vi "Parse Elements Treewise.vi"(6 "VI Refs":refnum<vi>[](array[refnum]), 7 "VI Data in":T3[](array[typedef]), 8 "error in":errorcluster, 9 "Parents":string[](array[string]), 10 "XML Info":T2, 11 "Node in":refnum<k20>) -> (0 "error out":errorcluster, 3 "Node out":refnum<k20>, 4 "VI Refs out":refnum<vi>[](array[refnum]), 5 "VI Data out":T3[](array[typedef]))   [LabVIEW 2020, in "VI Properties Editor.lvlib"]
uses:
  VI Properties Editor.lvlib
  <vilib>/xml/NI_XML.lvlib
  <vilib>/xml/Close Reference(Node).vi
  CTLs/XPath Get Attribute.ctl
  <vilib>/picture/picture.llb/imagedata.ctl
  CTLs/VI Properties.ctl
  CTLs/Control Properties.ctl
  CTLs/VI Data.ctl
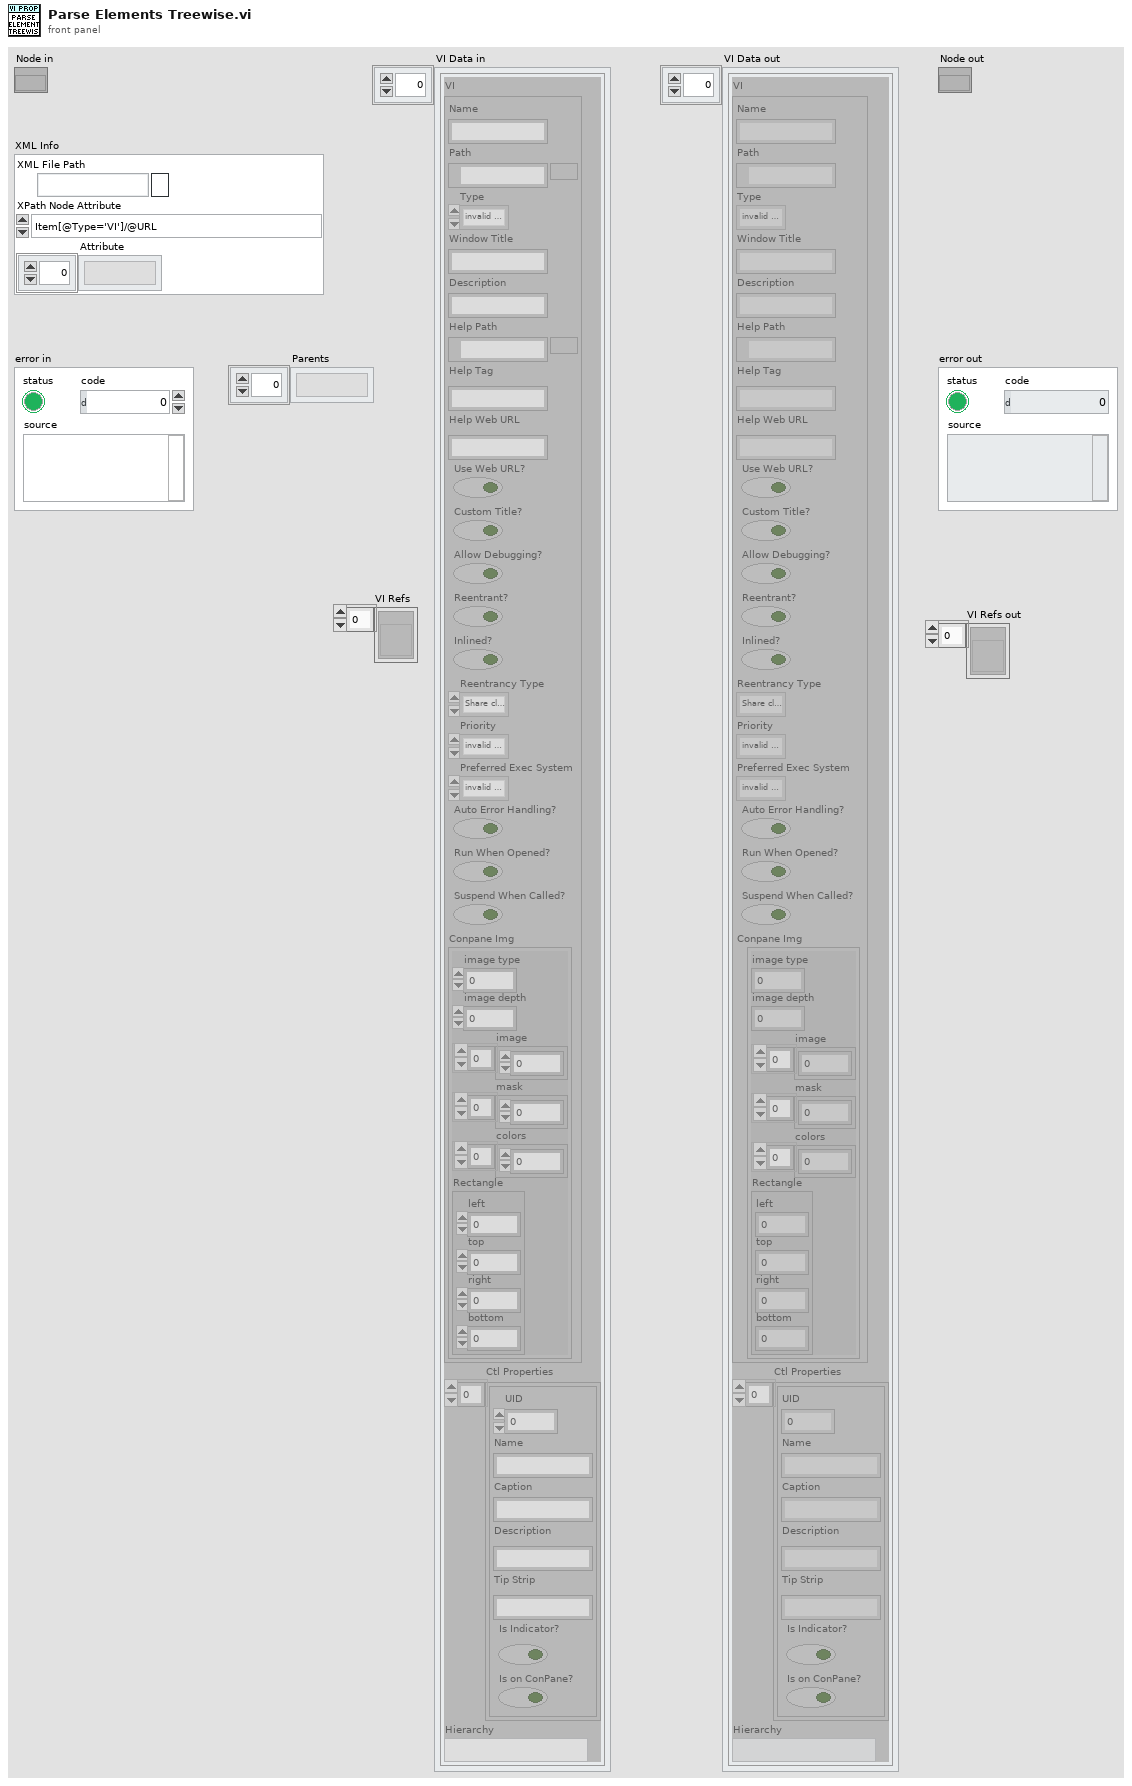
[diagram p1: front panel]
types:
  T1 = typedef "VI Properties Editor.lvlib/XPath Get Attribute.ctl" = enum16{"Item[@Type='VI']/@URL", "Item[@Type='LVClass']/@URL", "Item[@Type='Library']/@URL", "Item[@Type='Folder' and not (@URL)]/@Name", "@Name"}
  T2 = cluster{"XML File Path":path, "XPath Node Attribute":T1, "Attribute":string[]}
  T3 = typedef "VI Properties Editor.lvlib/VI Data.ctl" = cluster{"VI":T4, "Ctl Properties":T6[], "Hierarchy":string}
  T4 = typedef "VI Properties Editor.lvlib/VI Properties.ctl" = cluster{"Name":string, "Path":path, "Type":enum32{"invalid VI type", "Standard VI", "Control VI", "Global VI", "Polymorphic VI", "Configuration VI", "SubSystem", "Facade VI", "Method VI", "Statechart Diagram VI"}, "Window Title":string, "Description":string, "Help Path":path, "Help Tag":string, "Help Web URL":string, "Use Web URL?":bool, "Custom Title?":bool, "Allow Debugging?":bool, "Reentrant?":bool, "Inlined?":bool, "Reentrancy Type":enum16{"Share clones between instances", "Preallocate clone for each instance"}, "Priority":enum32{"invalid priority", "background priority", "normal priority", "above normal priority", "high priority", "time critical priority", "subroutine"}, "Preferred Exec System":enum32{"invalid execution system", "user interface", "standard", "instrument i/o", "data acquisition", "other 1", "other 2", "same as caller"}, "Auto Error Handling?":bool, "Run When Opened?":bool, "Suspend When Called?":bool, "Conpane Img":T5}
  T5 = typedef "imagedata.ctl" = cluster{"image type":i32, "image depth":i32, "image":u8[], "mask":u8[], "colors":u32[], "Rectangle":cluster{"left":i16, "top":i16, "right":i16, "bottom":i16}}
  T6 = typedef "VI Properties Editor.lvlib/Control Properties.ctl" = cluster{"UID":i32, "Name":string, "Caption":string, "Description":string, "Tip Strip":string, "Is Indicator?":bool, "Is on ConPane?":bool}
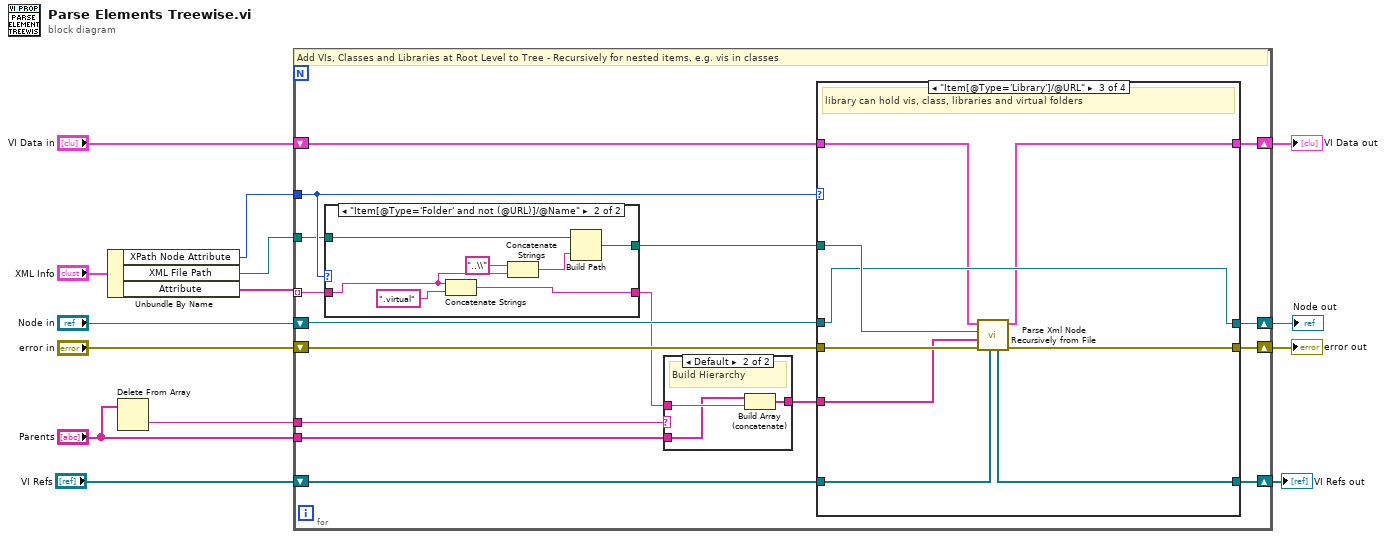
[diagram p0: block diagram]
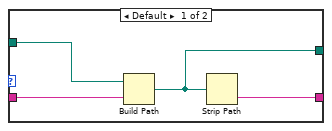
[diagram p2: hidden frame]
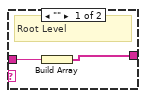
[diagram p3: hidden frame]
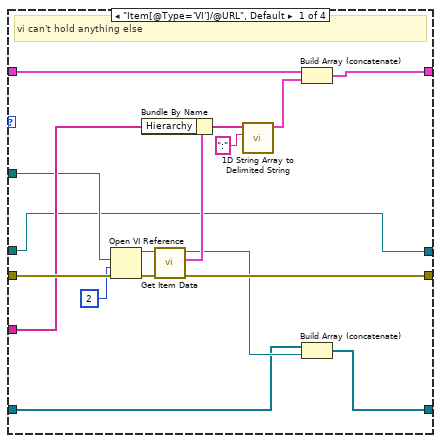
[diagram p4: hidden frame]
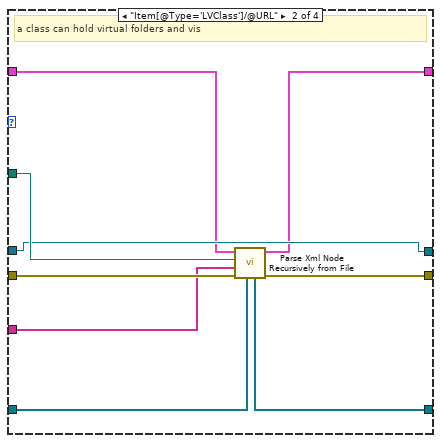
[diagram p5: hidden frame]
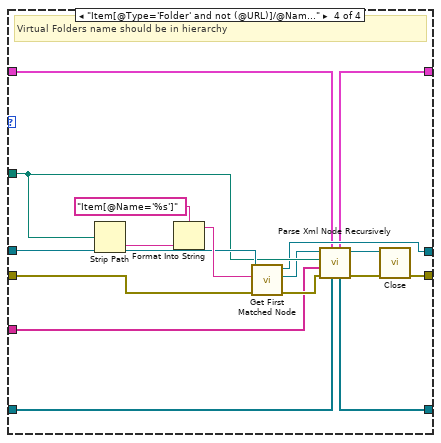
[diagram p6: hidden frame]
diagram:
  n1 = Unbundle By Name("XML Info") -> ("XPath Node Attribute"=w4:T1, "XML File Path"=w5:path, "Attribute"=w3:string[])
  n2 = Delete From Array(array="Parents") -> (deleted portion=w8:string)  [unwired: 2 in, 1 out]
  n3 = for {
    shift-right: [w30] -> w10
    shift-left: "error in" -> [w24]
    tunnel: w4 -> [w22]
    tunnel: w5 -> [w19]
    tunnel: w3 -> [w20] mode=indexing
    tunnel: "Parents" -> [w25]
    shift-right: [w28] -> w13
    shift-left: "VI Data in" -> [w27]
    tunnel: w8 -> [w26]
    shift-right: [w17] -> w7
    shift-left: "Node in" -> [w23]
    shift-right: [w15] -> w1
    shift-left: "VI Refs" -> [w16]
    # "Add VIs, Classes and Libraries at Root Level to Tree - Recursively for nested items, e.g. vis in classes"
    n4 = case shown="\"Item[@Type='Folder' and not (@URL)]/@Name\"" w22 {
      tunnel: w20 -> [w33 w39]
      tunnel: [w32 w40] -> w21
      tunnel: w19 -> [w34 w37]
      tunnel: [w31 w35] -> w18
      frame Default {
        n5 = Build Path(base path=w34, name or relative path=w33) -> (appended path=w31:path)
        n6 = Strip Path(path=w31) -> (name=w32:string)  [unwired: 1 out]
      }
      frame "Item[@Type='Folder' and not (@URL)]/@Name" {
        # "Virtual F."
        n7 = Concatenate Strings(w39, ".virtual" ("string")) -> (w40:string)
        n8 = Concatenate Strings("..\\" ("string"), w39) -> (w36:string)
        n9 = Build Path(base path=w37, name or relative path=w36) -> (appended path=w35:path)
      }
    }
    n10 = case shown="Default" w26 {
      tunnel: w21 -> [w43 w46]
      tunnel: [w42 w45] -> w29
      tunnel: w25 -> [_ w44]
      frame "" {
        # "Root Level"
        n11 = Build Array(w43) -> (w42:string[])
      }
      frame Default {
        # "Build Hierarchy"
        n12 = Build Array (concatenate)(w44, w46) -> (w45:string[])
      }
    }
    n13 = case shown="\"Item[@Type='Library']/@URL\"" w22 {
      tunnel: [w63 w72 w80 w97] -> w30
      tunnel: w24 -> [w62 w71 w81 w93]
      tunnel: w18 -> [w51 w70 w79 w91]
      tunnel: w29 -> [w57 w69 w78 w86]
      tunnel: [w52 w66 w75 w84] -> w28
      tunnel: w27 -> [w56 w67 w76 w85]
      tunnel: w23 -> [w50 w68 w77 w94]
      tunnel: [w50 w68 w77 w87] -> w17
      tunnel: w16 -> [w48 w65 w74 w83]
      tunnel: [w47 w64 w73 w82] -> w15
      frame "Item[@Type='VI']/@URL", Default {
        # "vi can't hold anything else"
        n14 = Open VI Reference(vi path=w51, options=2, error in (no error)=w62) -> (vi reference=w60:refnum<vi>, error out=w61:errorcluster)  [unwired: 3 in]
        n15 = call "Get Item Data.vi"("error in (no error)"=w61, "VI Ref"=w60) -> ("error out"=w63:errorcluster, "VI Data"=w55:T3, "VI Ref out"=w49:refnum<vi>)  [unwired: 7 in]
        n16 = call <vilib>:"1D String Array to Delimited String.vi"("delimiter"=":", "string array"=w57) -> ("delimited string"=w53:string)  [unwired: 9 in]
        n17 = Bundle By Name(cluster=w55, "Hierarchy"=w53) -> (w54:T3)
        n18 = Build Array (concatenate)(w56, w54) -> (w52:T3[])
        n19 = Build Array (concatenate)(w48, w49) -> (w47:refnum<vi>[])
      }
      frame "Item[@Type='LVClass']/@URL" {
        # "a class can hold virtual folders and vis"
        n20 = call "Parse Xml Node Recursively from File.vi"("VI Refs"=w65, "error in"=w71, "Parents"=w69, "Path to XML document"=w70, "VI Data"=w67) -> ("error out"=w72:errorcluster, "VI Data out"=w66:T3[], "VI Refs out"=w64:refnum<vi>[])  [unwired: 4 in]
      }
      frame "Item[@Type='Library']/@URL" {
        # "library can hold vis, class, libraries and virtual folders"
        n21 = call "Parse Xml Node Recursively from File.vi"("VI Refs"=w74, "error in"=w81, "Parents"=w78, "Path to XML document"=w79, "VI Data"=w76) -> ("error out"=w80:errorcluster, "VI Data out"=w75:T3[], "VI Refs out"=w73:refnum<vi>[])  [unwired: 4 in]
      }
      frame "Item[@Type='Folder' and not (@URL)]/@Name" {
        # "Virtual Folders name should be in hierarchy"
        n22 = Strip Path(path=w91) -> (name=w90:string)  [unwired: 1 out]
        n23 = Format Into String(format string="Item[@Name='%s']" ("XPath expression"), w90) -> (resulting string=w95:string)  [unwired: 2 in, 1 out]
        n24 = call <vilib>:"Get First Matched Node.vi"("error in (no error)"=w93, "XPath expression"=w95, "node in"=w94) -> ("error out"=w92:errorcluster, "node result"=w89:refnum<k20>, "node out"=w87:refnum<k20>)  [unwired: 6 in]
        n25 = call "Parse Xml Node Recursively.vi"("VI Refs"=w83, "VI Data"=w85, "error in"=w92, "Parents"=w86, "XML File Path"=w91, "Node in"=w89) -> ("error out"=w98:errorcluster, "Node out"=w88:refnum<k20>, "VI Refs out"=w82:refnum<vi>[], "VI Data out"=w84:T3[])  [unwired: 2 in]
        n26 = call-poly <vilib>:"Close.vi"("error in (no error)"=w98, "node"=w88) -> ("error out"=w97:errorcluster)  [unwired: 7 in]
      }
    }
  }
  "VI Data out" <- w13
  "error out" <- w10
  "Node out" <- w7
  "VI Refs out" <- w1
